vi "svfa_Compute Cross Spectrum.vi"(2 "sampling frequency [Hz]":dbl=10000.0 format="%.2f", 3 "signal Y [EUy]":dbl[](array[numeric]) format="%.2f", 4 "signal X [EUx]":dbl[](array[numeric]) format="%.2f") -> (0 "df [Hz]":dbl format="%.2f", 1 "cross spectrum [EUx EUy rms]":cdb[](array[numeric]) format="%.2f")   [LabVIEW 2017]
uses:
  <vilib>/Analysis/2dsp.llb/Cross Power (DBL).vi
  <vilib>/Analysis/NI_AALPro.lvlib
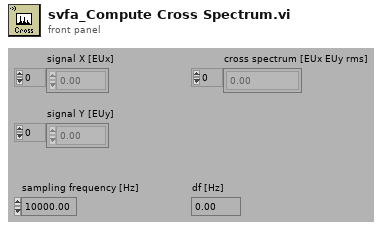
[diagram p1: front panel]
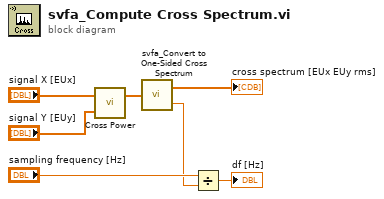
[diagram p0: block diagram]
diagram:
  n1 = call-poly <vilib>:"Cross Power.vi"("Y"="signal Y [EUy]", "X"="signal X [EUx]") -> ("Sxy"=w3:cdb[])  [unwired: 1 out]
  n2 = call <vilib>:"svfa_Convert to One-Sided Cross Spectrum.vi"("two-sided cross spectrum"=w3) -> ("one-sided cross spectrum"=→"cross spectrum [EUx EUy rms]":cdb[], "block size"=w1:dbl)
  n3 = Divide(x="sampling frequency [Hz]", y=w1) -> (x/y=→"df [Hz]":dbl)
